vi "z_scan_write.vi"(11 "address in":u32) -> (0 "FIFO scan time out":bool, 3 "address out":u32)   [LabVIEW 2010]
uses:
  <vilib>/rvi/DataTransferAndStorage/Container/XNode/niFpgaContainer.xnode
  <vilib>/rvi/DataTransferAndStorage/Container/Common/niFpgaContainerMethod.ctl
  <vilib>/rvi/DataTransferAndStorage/Container/Common/niFpgaTransferTypeControl.ctl
  <vilib>/rvi/interface/RandomDataEmulation/nirviRandomDataFPGAFIFO.vi
  <vilib>/rvi/interface/RandomDataEmulation/niFpgaRandomDataHandleErrors.vi
  <vilib>/rvi/Memory/Memory_Emulation/nirvimemoryEmulationManagerCache_GetValue.vi
  <vilib>/rvi/DataTransferAndStorage/Container/Common/niFpgaContainerGetUniqueNameForEmu.vi
  <vilib>/rvi/Memory/Memory_Emulation/nirvimemoryEmulationManagerCache_InsertValue.vi
  <vilib>/Utility/error.llb/Clear Errors.vi
  <vilib>/rvi/Memory/Memory_Emulation/nirvimemoryEmulationManagerCache_SetValue.vi
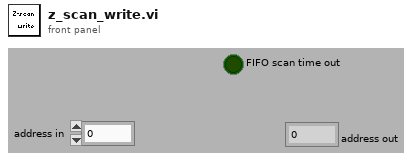
[diagram p1: front panel]
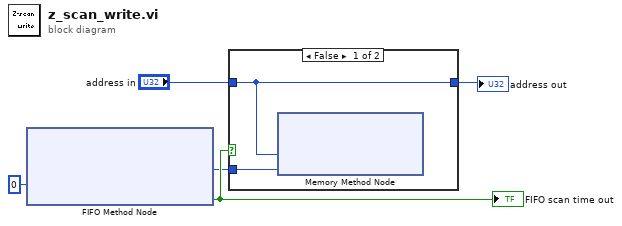
[diagram p0: block diagram]
diagram:
  n1 = xnode ("FIFO Method Node")("Timeout"=0) -> ("Element"=w1:u32, "Timed Out?"=w2:bool)  [unwired: 1 in, 1 out]
  "FIFO scan time out" <- w2
  n2 = case shown="False" w2 {
    tunnel: "address in" -> [w6 w133]
    tunnel: [w6 w133] -> w4
    tunnel: w1 -> [w7 _]
    frame False {
      n3 = xnode ("Memory Method Node")("Address"=w6, "Data"=w7) -> ()  [unwired: 1 in, 1 out]
    }
    frame True {
    }
  }
  "address out" <- w4
